vi "20_ВПРегистр.vi"() -> ()   [LabVIEW 2016]
panel:
  in  "stop":bool
  out "Отсчёт 3 итерации назад":dbl
  out "Отсчёт 2 итерации назад":dbl
  out "Предыдущий отсчёт":dbl
  out "Текущий отсчёт":dbl
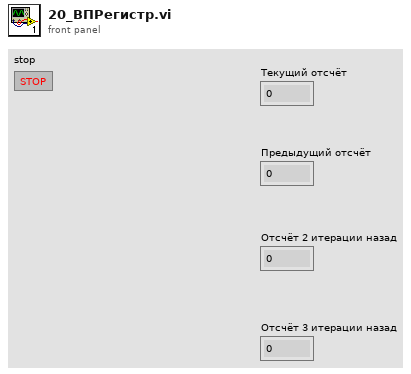
[diagram p1: front panel]
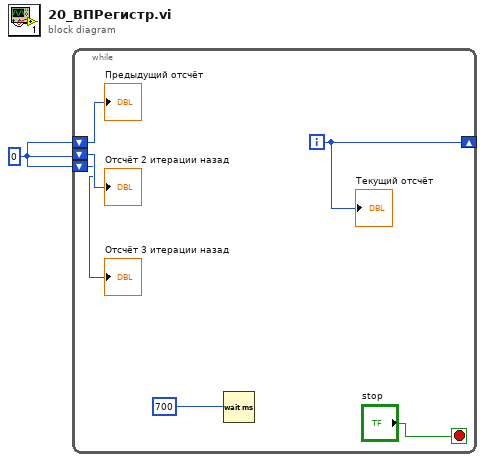
[diagram p0: block diagram]
diagram:
  w1 = 0
  n1 = while {
    shift-right: [w3] -> _
    shift-left: w1 -> [w6]
    shift-left: w1 -> [w5]
    shift-left: w1 -> [w4]
    i -> [w3]
    stop <- "stop" stop-if-true
    n2 = Wait (ms)(milliseconds to wait=700) -> ()  [unwired: 1 out]
    "Текущий отсчёт" <- w3
    "Предыдущий отсчёт" <- w6
    "Отсчёт 2 итерации назад" <- w5
    "Отсчёт 3 итерации назад" <- w4
  }
